vi "Sandbox.vi"() -> ()   [LabVIEW 2020, in "Sandbox.lvlib"]
uses:
  Sandbox.lvlib
  <vilib>/gpm_packages/@cs/Configuration/Source/ConfigurationReference/ConfigurationReference.lvclass/ConfigurationReference.ctl
  5cb79e3e-957d-4d32-824f-023e3e129628.vi
  a327098c-d06f-4deb-a132-a30ee28da86d.vi
  <vilib>/gpm_packages/@cs/Configuration/Source/ConfigurationReference/Explain DVR Error.vi
  5cb79e3e-957d-4d32-824f-023e3e129628.vi/8402ebc0-384b-46ab-989c-700e41096983.vi
  <vilib>/gpm_packages/@cs/Configuration/Source/ConfigurationReference/Read IConfiguration.vi
  <vilib>/gpm_packages/@cs/Configuration/Source/ConfigurationReference/Write IConfiguration.vi
  a327098c-d06f-4deb-a132-a30ee28da86d.vi/7595dcc0-0a31-43e1-86ad-579fe37a7e85.vi
  <vilib>/gpm_packages/@cs/Configuration/Source/IConfiguration/Write U64.vi
  <vilib>/gpm_packages/@cs/Configuration/Source/IConfiguration/Read U64.vi
  Source/mysql-queries/mysql-queries.lvclass
  C:/Users/Fred.Guo/Desktop/Database-configuration/Source/IConfigDBQueries/IConfigurationDatabaseQueries.lvclass
  externals/mysql/Source/mysql.net/mysql.lvclass
  C:/Users/Fred.Guo/Desktop/Database-configuration/externals/database-interface/Source/IDatabase/IDatabase/IDatabase.lvclass
  Source/configuration-database.lvclass
  C:/Program Files/National Instruments/LabVIEW 2020/vi.lib/gpm_packages/@cs/Configuration/Source/IConfiguration/IConfiguration.lvclass
  <vilib>/gpm_packages/@cs/Configuration/Source/IConfiguration/IConfiguration.lvclass
  <vilib>/gpm_packages/@cs/Configuration/Source/ConfigurationReference/ConfigurationReference.lvclass
  C:/Users/Fred.Guo/Desktop/Database-configuration/externals/database-interface/IDatabase/IDatabase/IDatabase.lvclass
  C:/Users/Fred.Guo/Desktop/Database-configuration/externals/mysql/Source/mysql.net/mysql.lvclass
  C:/Users/Fred.Guo/Desktop/Database-configuration/Source/mysql-queries/mysql-queries.lvclass
  C:/Users/Fred.Guo/Desktop/Database-configuration/Source/configuration-database.lvclass
panel:
  in  "ItemName":string="Boop"
  out "Great success?":bool
  in  "Value":u64=123
  out "Not Found?":bool
  out "error out":errorcluster
  out "Value":u64
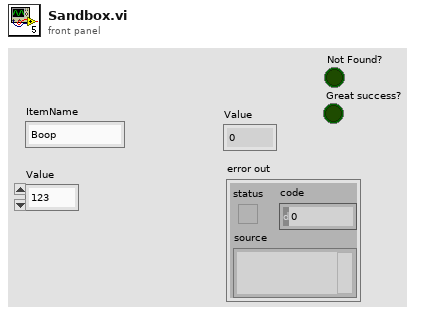
[diagram p1: front panel]
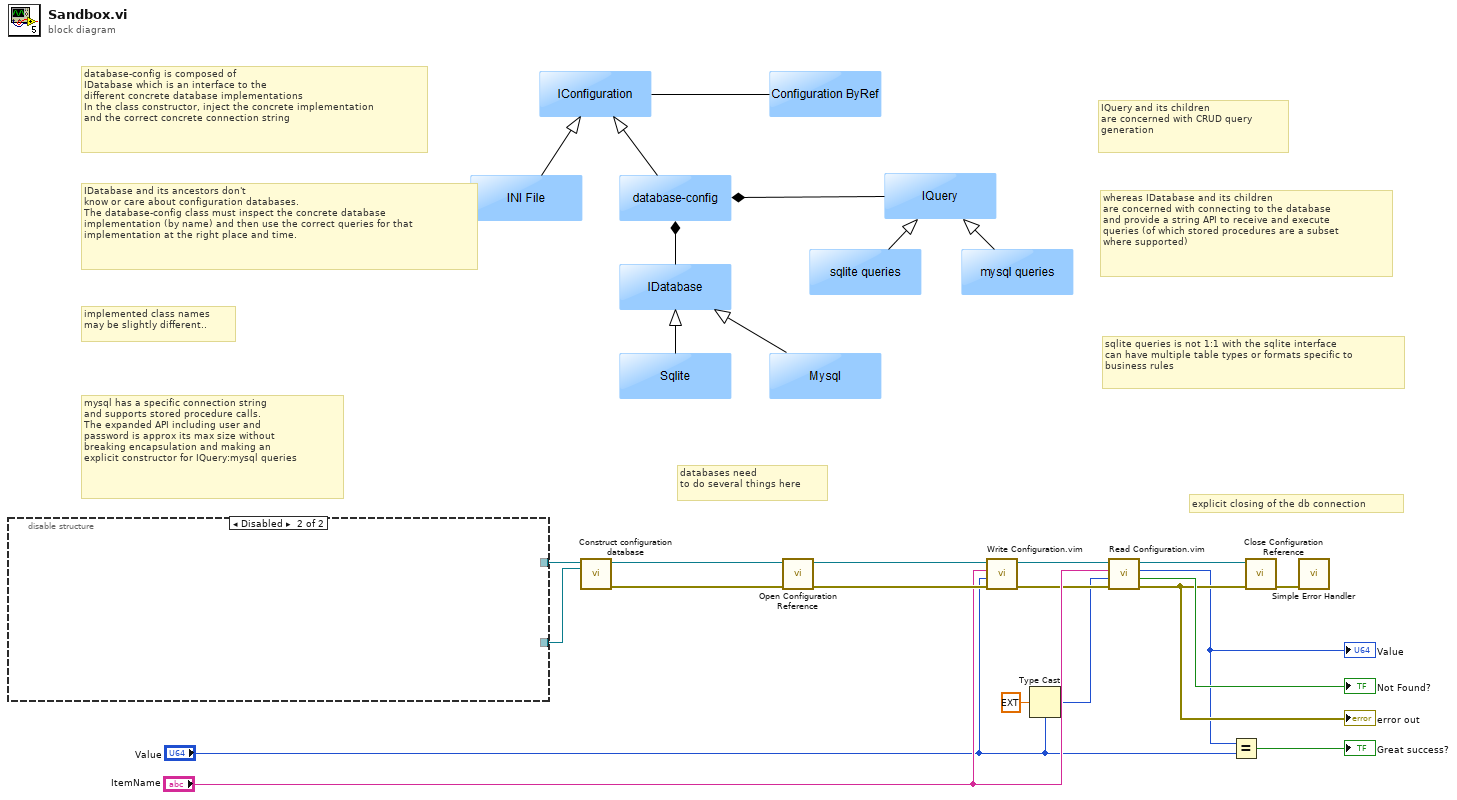
[diagram p0: block diagram]
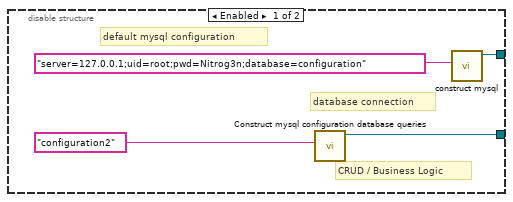
[diagram p2: hidden frame]
diagram:
  # "sqlite queries is not 1:1 with the sqlite interface\ncan have multiple table types or formats specific to\nbusiness rules"
  # "explicit closing of the db connection"
  # "databases need\nto do several things here"
  # "whereas IDatabase and its children\nare concerned with connecting to the database\nand provide a string API to receive and execute\nqueries (of which stored procedures are a subset\nwhere supported)"
  # "IQuery and its children\nare concerned with CRUD query\ngeneration"
  # "implemented class names\nmay be slightly different.."
  # "IDatabase and its ancestors don't \nknow or care about configuration databases.\nThe database-config class must inspect the concrete database\nimplementation (by name) and then use the correct queries for that\nimplementation at the right place and time."
  # "mysql has a specific connection string\nand supports stored procedure calls.\nThe expanded API including user and \npassword is approx its max size without\nbreaking encapsulation and making an\nexplicit constructor for IQuery:mysql queries"
  # "database-config is composed of \nIDatabase which is an interface to the\ndifferent concrete database implementations\nIn the class constructor, inject the concrete implementation\nand the correct concrete connection string"
  n1 = disable-structure shown="Disabled" {
    disable-tunnel: [w20 _] -> w2
    disable-tunnel: [w19 _] -> w1
    frame Enabled {
      # "CRUD / Business Logic"
      # "database connection"
      # "default mysql configuration"
      n2 = call "Construct mysql configuration database queries.vi"("table"="configuration2" ("table name (configuration)")) -> ("mysql-configdb-queries out"=w19:refnum<class "mysql-queries.lvclass">)  [unwired: 9 in, 1 out]
      n3 = call "construct mysql.vi"("Connection string"="server=127.0.0.1;uid=root;pwd=Nitrog3n;database=configuration" ("Name")) -> ("mysql out"=w20:refnum<class "mysql.lvclass">)  [unwired: 9 in, 1 out]
    }
    frame Disabled {
    }
  }
  n4 = call "Construct configuration database.vi"("SQL logic type"=w1, "Database type in"=w2) -> ("error out"=w10:errorcluster, "database-configuration out"=w11:refnum<class "configuration-database.lvclass">)  [unwired: 8 in]
  n5 = call <vilib>:"Open Configuration Reference.vi"("error in (no error)"=w10, "Configuration Type"=w11) -> ("error out"=w13:errorcluster, "Configuration Reference"=w14:refnum<data-value>)  [unwired: 8 in]
  n6 = call "Write Configuration.vim"("error in (no error)"=w13, "Value"="Value", "Name"="ItemName", "Configuration Reference in"=w14) -> ("error out"=w6:errorcluster, "Configuration Reference out"=w7:refnum<data-value>)  [unwired: 6 in]
  n7 = Type Cast(type="Value", x=ext 0.0) -> (*(type *) &x=w4:u64)
  n8 = call "Read Configuration.vim"("error in (no error)"=w6, "Type (Default Value If Not Found)"=w4, "Name"="ItemName", "Configuration Reference in"=w7) -> ("error out"=w16:errorcluster, "Not Found?"=→"Not Found?":bool, "Value"=w9:u64, "Configuration Reference out"=w17:refnum<data-value>)  [unwired: 4 in]
  "Value" <- w9
  "error out" <- w16
  n9 = Equal?(x=w9, y="Value") -> (x = y?=→"Great success?":bool)
  n10 = call <vilib>:"Close Configuration Reference.vi"("error in (no error)"=w16, "Configuration Reference"=w17) -> ("error out"=w15:errorcluster)  [unwired: 9 in]
  n11 = call <vilib>:"Simple Error Handler.vi"("error in (no error)"=w15) -> ()  [unwired: 4 in, 5 out]
